vi "Individual curve visualization-Original.vi"() -> ()   [LabVIEW 2016]
panel:
  out "Drag V 4":cluster{dbl[], "Drag R":dbl[]}(graph)={[1.0, 1.2, 1.4, 1.6, 1.8, 2.0, 2.2, 2.4000000000000004, 2.6, 2.8, 3.0, 3.2, 3.4000000000000004, 3.6, 3.8000000000000003, 4.0, 4.2, 4.4, 4.6, 4.800000000000001, 5.0, 5.2, 5.4, 5.6000000000000005, 5.800000000000001, 6.0, 6.2, 6.4, 6.6000000000000005, 6.800000000000001, 7.0, 7.2, 7.4, 7.6000000000000005, 7.800000000000001, 8.0, 8.2, 8.4, 8.600000000000001, 8.8, 9.0], "Drag R"=[-3.300713023076663, -3.154449474386773, -1.6018811853832888, -1.623056110644585, -2.807731924651278, -4.278396429154972, -4.279502183141707, -4.366286193642124, -1.4410534649772644, 0.15566028543242932, 1.6991261140725915, 1.5692536155403247, 2.8580510224343625, 1.8206622631926488, 1.065024446971932, 0.32155007033235866, 0.4290224922843568, -0.6739053828926125, -1.9963504895407167, -1.9615097922476261, -3.7035483297953604, -2.7529582838595164, -3.432489372671602, -2.673522191757494, -3.4326797147495465, -4.140057534177399, -4.516110550482156, -6.970872132203194, -8.198832275397276, -5.3032397571211645, -3.8902609432575925, -5.869261674603283, -9.2239063545535, -6.918059763808269, -7.5433263379328475, -5.669627470898903, -6.863865171357286, -6.912037847582487, -5.835029601349728, -6.006897427720724, -7.171526427705753]}
  out "Drag V 2":cluster{dbl[], "Drag R":dbl[]}(graph)={[-1.0, -1.2, -1.4, -1.6, -1.8, -2.0, -2.2, -2.4000000000000004, -2.6, -2.8, -3.0, -3.2, -3.4000000000000004, -3.6, -3.8000000000000003, -4.0, -4.2, -4.4, -4.6, -4.800000000000001, -5.0, -5.2, -5.4, -5.6000000000000005, -5.800000000000001, -6.0, -6.2, -6.4, -6.6000000000000005, -6.800000000000001, -7.0, -7.2, -7.4, -7.6000000000000005, -7.800000000000001, -8.0, -8.2, -8.4, -8.600000000000001, -8.8, -9.0], "Drag R"=[-3.2437419601821214, -3.0741664524350005, -1.6279568878167145, -1.6200422715203617, -2.6283908576894714, -3.888715770646895, -3.977618456971424, -4.319620743435273, -1.3664134385707647, 0.320047182291161, 1.7072885590830775, 1.7630417095507562, 3.480405410849366, 1.8585977537912803, 1.1069080457471894, 0.19196943000107664, 0.36263224393675075, -0.5459969964599499, -2.246495774976516, -1.9887416826811497, -3.328699227235056, -2.8303882648843945, -3.046031238207835, -3.1669715718770597, -2.935142589811789, -4.499040388432356, -4.461115990090428, -6.5530890706250915, -7.938589412259593, -4.850132199040752, -3.8820527919237495, -5.861039921112386, -8.632298570084401, -6.880111107470923, -7.4081336329075675, -5.545023198155025, -6.610745934318789, -6.902518778616165, -5.879443445946976, -5.861498347694719, -7.106378902925503]}
  out "Drag V 3":cluster{dbl[], "Drag R":dbl[]}(graph)={[-1.0, -1.2, -1.4, -1.6, -1.8, -2.0, -2.2, -2.4000000000000004, -2.6, -2.8, -3.0, -3.2, -3.4000000000000004, -3.6, -3.8000000000000003, -4.0, -4.2, -4.4, -4.6, -4.800000000000001, -5.0, -5.2, -5.4, -5.6000000000000005, -5.800000000000001, -6.0, -6.2, -6.4, -6.6000000000000005, -6.800000000000001, -7.0, -7.2, -7.4, -7.6000000000000005, -7.800000000000001, -8.0, -8.2, -8.4, -8.600000000000001, -8.8, -9.0], "Drag R"=[8.506268720241243, 8.453111299769647, 5.837640325861369, 7.148519535853817, 5.613151260951883, 7.15271594863945, 6.035303430479679, 4.099468581977172, 3.8085835691967307, 2.146728062452322, 2.5912692993997513, 3.2852570243268238, 6.045815515529311, 5.520600455246357, 9.329259679090598, 10.480605588956307, 7.047030330219627, 8.091806546725207, 12.243345671940846, 13.329586545967194, 9.70803891981146, 10.868730098486818, 11.122912960745628, 10.009136477603038, 9.624346942261845, 8.817803908300313, 9.52354730833524, 6.612316030305441, 4.372195049370224, 2.659259797064494, 1.5932641526471045, 1.3933543185710036, 4.119548088345109, 5.4968037601237425, 6.930305725770583, 5.8104621629971245, 6.426504856124536, 6.12416493376701, 6.3797355980905195, 7.247784092040921, 6.868995388580276]}
  out "Drag R from V3":dbl[][](graph)=[[100.0], [100.0], [100.0], [100.0], [100.0], [100.0], [100.0], [100.0], [100.0], [100.0], [100.0], [100.0], [1.7525787802191088], [1.7024277791309896], [1.6796467941372961], [1.6622332596780016], [1.6326384430038565], [1.6030538217028973], [1.5750233368612336], [1.5464672130079027], [1.515305674671948], [1.4769663724594069], [1.4223433405393917], [1.367127876528625], [1.3303848800977325], [1.3258115595086495], [1.3319441343876612], [1.3412111211499946], [1.3504840018871018], [1.3569460556411512], [1.3612603273002564], [1.3655187586981927], [1.3717149148393943], [1.3853607545603541], [1.4256734959642343], [1.4882323948260159], [1.5646664564337707], [1.6600043991998266], [1.825179103810554], [2.0113113690130784], [2.153778457836145], [2.2061854757169623], [2.236759390639608], [2.2591165259970976], [2.271254546163343], [2.255116888990723], [2.131284142338929], [1.9300209107430364], [1.6997469455502165], [1.4689595661227408], [1.1719038462170055], [0.8507746640096665], [0.5682848756976853], [0.36799449880168633], [0.18504407697053282], [0.030652355361287242], [-0.06621522446930839], [-0.0895003694716015], [-0.09847025618305347], [-0.10464033846391654], [-0.10781778022866328], [-0.09364334174838697], [0.005606370088155135], [0.15965049598821562], [0.3473966553463515], [0.6442898471825012], [0.9527207762518782], [1.1676473220636312], [1.3374546714193756], [1.478434752127217], [1.5901322848992354], [1.6761660916131926], [1.7571344209049884], [1.8539291022681812], [1.9672049616575058], [2.084724071244043], [2.1942627160586827], [2.286993956635236], [2.37381081162657], [2.4528785475558], [2.5192696643991765], [2.570526739598677], [2.616689286852219], [2.6556743975271786], [2.682945368739358], [2.6962103781729607], [2.7059545183791447], [2.713853497772562], [2.719510645535571], [2.7225292908505287], [2.710925280793093], [2.6300724971380625], [2.507075147000063], [2.382324413515172], [2.284609434023482], [2.17962607717798], [2.0831734899557364], [2.022088082940096], [2.013507711742533], [2.0156321567498408], [2.0189057281954095], [2.022310702355015], [2.024991414457769], [2.0273587980551864], [2.029723297463262], [2.03228399843974], [2.0350593304874858], [2.037491663799248], [2.0404356617865664], [2.0449630021118885], [2.0589709240612515], [2.1147157107984738], [2.1951299818846985], [2.2809633053678966], [2.3878215220763006], [2.5123411459049585], [2.646121499165556], [2.7849929260300934], [2.94150608367427], [3.1001579479531576], [3.2446358461914926], [3.3828302948475217], [3.510267351861236], [3.6279185045827487], [3.738281105160597], [3.752281712877838], [3.716968130527663], [3.668561387705247], [3.6302480115875677], [3.619709418125278], [3.6170633689313596], [3.614338362318714], [3.6039982532236], [3.5632666463112197], [3.496188667064237], [3.4112673848251758], [3.302064135284801], [3.113108995158534], [2.9035833460838285], [2.7395191524712423], [2.6003692519174293], [2.470750349283642], [2.342683551892261], [2.2113055620953066], [2.084513208934559], [1.9502420264794773], [1.7841432231673235], [1.5808808468002922], [1.4589808708783767], [1.386113150959947], [1.3097468509102916], [1.2294193993280012], [1.3183489806063184], [1.7735900985853585], [1.8434364938950272], [1.6547838114359072], [1.4438849144543546], [1.1713380909804658], [0.9591404583844942], [0.9332570698213668], [0.9796520082449389], [1.0260469466685094], [1.0324380863668592], [1.0211745682940934], [1.0041594665245963], [0.9871443647550996], [0.9758808466823338], [0.9776632604651697], [1.0017554362928947], [1.0407717416081217], [1.0851455193601809], [1.1253101124984026], [1.1548084930482103], [1.1846991314501096], [1.2135526797068725], [1.2370487555268035], [1.250866976618206], [1.250745581339546], [1.2356121483481992], [1.2086064106811254], [1.1731312848415776], [1.132589687332811], [1.09038453465808], [1.0486634617941106], [1.001886957066429], [0.9485974335154795], [0.8884358369283974], [0.8210431130923201], [0.7460602077943783], [0.6601291617269677], [0.5483458064502711], [0.41616454664051356], [0.2724218383288142], [0.12595413754630536], [-0.014402099675880353], [-0.143103745292994], [-0.2729409413039015], [-0.40314083661617306], [-0.5298446554967583], [-0.6491936222126193], [-0.757328961030706], [-0.8530136281214128], [-0.9476966326108381], [-1.039060936123331], [-1.1221208120951789], [-1.19189053396267], [-1.2433843751620999], [-1.274731627175126], [-1.301236592248865], [-1.3251172476858604], [-1.3456543216920223], [-1.362128542473259], [-1.3738206382354787], [-1.3800113371845906], [-1.3804558837599505], [-1.3779361904824217], [-1.373879057238943], [-1.3693094440068145], [-1.3652523107633359], [-1.3627326174858072], [-1.3650331323236395], [-1.38469300364413], [-1.4198004223987497], [-1.4659599201843385], [-1.5187760285977352], [-1.573853279235783], [-1.626796203695321], [-1.6769446709488391], [-1.740232688366131], [-1.8106780565794993], [-1.8783318445699293], [-1.9332451213184072], [-1.965468955805924], [-1.9678038585291104], [-1.9512967158820373], [-1.920245912954881], [-1.8767003009131922], [-1.8227087309225247], [-1.7603200541484314], [-1.6915831217564676], [-1.6113302167838213], [-1.4819493743337553], [-1.3075715032524697], [-1.099948368593185], [-0.8708317354091007], [-0.6319733687534363], [-0.39512503367941276], [-0.16457147591045432], [0.0923245398572996], [0.37022252797865973], [0.656269081742926], [0.9376107944394273], [1.2013942593574631], [1.434766069786344], [1.6335917384754741], [1.8370718061323112], [2.040408441631051], [2.2300560533477376], [2.392469049658433], [2.5141018389391805], [2.581408829566029], [2.587269792136006], [2.563182205515298], [2.5186136886096357], [2.4573277088998084], [2.3830877338666054], [2.2996572309908103], [2.210799667753213], [2.1137606212460303], [1.976290685287626], [1.8035435235688344], [1.6075345200211748], [1.4002790585761735], [1.1937925231653364], [1.000090297720189], [0.82260339531407], [0.6252364316180199], [0.4200976984206837], [0.22825713135653058], [0.07078466606002365], [-0.031249761834372003], [-0.06770993281922782], [-0.09095212558221256], [-0.11083457660248139], [-0.12715113040549347], [-0.13969563151670594], [-0.14826192446157663], [-0.1526438537655633], [-0.14512720156245154], [-0.0859364276435621], [0.018640823505575527], [0.1542000683837651], [0.30633682348982466], [0.46064660532255874], [0.6027249303807714], [0.7264653052044163], [0.8673965864580044], [1.0197838582519936], [1.1696103702022502], [1.3028593719246406], [1.405514113035026], [1.4635578431492866], [1.4713967826342518], [1.4708139625800953], [1.4696628267175604], [1.4679585099118064], [1.4657161470279927], [1.4629508729312792], [1.4596778224868248], [1.455912130559789], [1.4485516507878464], [1.4207008268694026], [1.3738396138374274], [1.3127644697521716], [1.242271852673886], [1.1671582206628266], [1.0922200317792337], [1.022253744083363], [0.959672974401438], [0.8939020095272481], [0.8246069275278078], [0.7537171894972365], [0.6831622565296582], [0.614871589719183], [0.550774650159935], [0.4928008989460335], [0.4428797971715981], [0.4013447226544859], [0.3603397198822643], [0.31966426780318175], [0.2806907156474203], [0.24479141264515478], [0.21333870802656751], [0.18770495102183835], [0.16926249086114714], [0.1593836767746737], [0.15886460367700045], [0.16482085143572592], [0.1760060038779972], [0.19166109431666914], [0.21102715606459688], [0.23334522243463546], [0.25785632673964], [0.2838015022924656], [0.3104217824059673], [0.3382548894224496], [0.3738794064184983], [0.41670200668102686], [0.4647834984216126], [0.516184689851833], [0.5689663891832655], [0.6211894046274875], [0.6709145443960733], [0.7168732647431969], [0.7618980836377554], [0.8066315567273659], [0.8511286828950316], [0.895444461023756], [0.9396338899965421], [0.9837519686963905], [1.0278536960063103], [1.0719940708093016], [1.116115336607255], [1.1597000030691473], [1.202956201549208], [1.2462163791241851], [1.2898129828708271], [1.3340784598658797], [1.379345257186097], [1.4256277248076368], [1.471485296017775], [1.5172787744285805], [1.5637021239542714], [1.611449308509066], [1.661214292007178], [1.7136910383628323], [1.7695735114902438], [1.8309839883668162], [1.9046172824357102], [1.9860303747238839], [2.0690664855450898], [2.147568835213081], [2.215380644041606], [2.2686544985483668], [2.3172066161165055], [2.362599182869531], [2.404320218709873], [2.441857743539961], [2.4746997772622246], [2.5023343397790923], [2.525058473852339], [2.5470074952941992], [2.567949852570494], [2.586821988927007], [2.6025603476095247], [2.6141013718638315], [2.620381504935713], [2.6178575569635028], [2.594543402738337], [2.557003662884257], [2.514722061153872], [2.477182321299792], [2.4538681670746265], [2.450996819724539], [2.4547599206884096], [2.461936852620605], [2.472163159873596], [2.485074386799855], [2.500306077751855], [2.517493777082067], [2.541823826637785], [2.600923739891003], [2.6864026626294564], [2.783728630273892], [2.8783696782450603], [2.955793841963711], [3.0014691568505936], [3.007738172514057], [3.0067715943183995], [3.0048540219622972], [3.0020017170477096], [2.9982309411765975], [2.9935579559509216], [2.987999022972642], [2.973414339278415], [2.904782397172163], [2.7839265288191064], [2.621259310737942], [2.427193319447388], [2.2121411314661588], [1.9865153233129669], [1.7481776221828689], [1.4370709950539666], [1.0634145232580363], [0.6505154137173521], [0.22168087335410447], [-0.199781890909434], [-0.5982712108318664], [-1.0035001233111378], [-1.4172115456511012], [-1.8341969688897715], [-2.249247884065137], [-2.6571557822152676], [-3.052712154378151], [-3.4398842877940368], [-3.8581720136922337], [-4.28510172470091], [-4.68787441313243], [-5.033691071299138], [-5.289752691513447], [-5.440350650806982], [-5.5662261660846895], [-5.679776400419057], [-5.777530122860715], [-5.856016102460291], [-5.911763108268416], [-5.941299909335716], [-5.936400757868801], [-5.871887982418222], [-5.756966412187664], [-5.606353244398619], [-5.434765676272584], [-5.256920905031052], [-5.078369089309328], [-4.859207835558015], [-4.605965162097498], [-4.334378641472833], [-4.060185846229073], [-3.799124348911274], [-3.5600243887590945], [-3.315477715068531], [-3.069965462792207], [-2.834687008697351], [-2.6208417295512425], [-2.439629002121144], [-2.2951588654826103], [-2.155543185831086], [-2.023482653164767], [-1.9087060191267227], [-1.8209420353599974], [-1.7699194535076614], [-1.7588434198871203], [-1.7546606014535835], [-1.7512727653155618], [-1.7487007891590096], [-1.7469655506698811], [-1.7460879275341306], [-1.751855458263503], [-1.7936825787784874], [-1.8640515659725108], [-1.94909954627763], [-2.0349636461259024], [-2.1107657071835297], [-2.1861503338360158], [-2.2645484000403884], [-2.3470281963582473], [-2.434658013351197], [-2.5285061415808414], [-2.633447831862587], [-2.76576525688769], [-2.9108401979112632], [-3.049399933779855], [-3.1621717433399823], [-3.2372201905266857], [-3.3041944651830177], [-3.363676754655715], [-3.4094562056991617], [-3.4353219650677413], [-3.4354093432619446], [-3.4100311479385788], [-3.3646864233529454], [-3.3050221253948866], [-3.2366852099542447], [-3.157410520087679], [-3.033190405000106], [-2.8817392207732864], [-2.7295521108014844], [-2.590179295629865], [-2.4313802714044446], [-2.3150918660558855], [-2.3130125039363834], [-2.425028818075278], [-2.606877496788717], [-2.8722725286059783], [-3.327858992828627], [-3.5688180648142787], [-3.7199668472843137], [-3.8101565478293744], [-3.765288778462918], [-3.409697192443322], [-2.96679199430353], [-2.6741029939543584], [-2.448920146122463], [-2.252319045044758], [-2.084091564551963], [-1.94537691470312], [-1.6968735048719377], [-1.293886787102919], [-1.4580039927133661], [-2.7229885215063963], [-3.728654949645486], [-4.525405046288279], [-4.639098086182561], [-4.46956993412352], [-4.208072423868329], [-3.902287561082815], [-3.4638730574051255], [-2.9985198915565334], [-2.5018614682929248], [-1.9869828598242254], [-1.4593775800740074], [-0.8707832293898149], [-0.3601316708142035], [-0.04943995450805877], [0.19629323636639384], [0.3507948582790463], [0.3380162987393554], [0.1161254986409278], [-0.17535228671281733], [-0.4025506122009139], [-0.6102714962103372], [-0.8010438345558084], [-0.9593066584794848], [-1.088135677620042], [-1.2063186055947464], [-1.3330973990654873], [-1.49370455119218], [-1.7053497458468536], [-1.8962169972012424], [-2.0017639876829647], [-2.076050790635698], [-2.1342272050896534], [-2.1774242008695355], [-2.206641323395504], [-2.224769072375174], [-2.2393187437991924], [-2.2582161776527747], [-2.291500907840678], [-2.3526117398782858], [-2.433266923925575], [-2.522274438668859], [-2.6176510564344566], [-2.750262465402251], [-2.884404748568754], [-2.9736990783630604], [-2.987016538674169], [-2.9868701783838003], [-2.9865783454859103], [-2.9861419662582533], [-2.979278268104357], [-2.9335910059997827], [-2.856354685647265], [-2.7617169585063355], [-2.656398344199613], [-2.5093599053719773], [-2.3257280117302135], [-2.117986853952131], [-1.8893782784491395], [-1.607550511810117], [-1.3028805487474227], [-0.9824579479639529], [-0.6354517643496308], [-0.579855452817553], [-0.6407153728110055], [-0.7437725343279338], [-0.9048365575977063], [-1.2553362874988296], [-1.6557051691660387], [-1.9557175645738285], [-2.2181944080310125], [-2.436394184721253], [-2.5910998420360447], [-2.73024945698041], [-2.8443994645533324], [-2.9118650897136553], [-2.9178661838259345], [-2.892982538232731], [-2.8501280690589894], [-2.796516155796167], [-2.7310891036650964], [-2.6204167857222087], [-2.4863979073377283], [-2.3602003525067876], [-2.2671538426013678], [-2.19014483701028], [-2.1206356877785804], [-2.0544544152560076], [-1.987020025520782], [-1.9162190383509248], [-1.8490026216374156], [-1.7932323558824346], [-1.7533642275345251], [-1.7180854727779578], [-1.6950700847375808], [-1.6974015702912149], [-1.7342024779298217], [-1.784616006204022], [-1.824445681719345], [-1.8353832658857139], [-1.8385671833127937], [-1.8412587788651278], [-1.8457017990214601], [-1.8518605983869163], [-1.8592343363340902], [-1.8674439269625895], [-1.8769720039864102], [-1.890856160010116], [-1.9050975063953381], [-1.9146405860914009], [-1.9102579085078448], [-1.8688279095700862], [-1.798925339458748], [-1.7140709923625235], [-1.6170415168737422], [-1.467181415798466], [-1.293560381117423], [-1.1371354262072777], [-1.0269245022843725], [-0.9240605507913129], [-0.8366322922367193], [-0.7837575427369969], [-0.7785726464057602], [-0.7954719089281913], [-0.8250141629137189], [-0.8627580820395703], [-0.9088427829311257], [-0.9843819487818842], [-1.0845884842201712], [-1.1998806677958647], [-1.324418201720993], [-1.473138994843593], [-1.6454955306516061], [-1.8374289898957854], [-2.0448805533269785], [-2.2637914016959293]]
  out "Drag R from V2":dbl[][](graph)
  out "Drag R from V1":dbl[][](graph)
  in  "Tab Control":enum32{"Drag R and 4T R", " Line cut"}(tab)=enum." Line cut"
  in  "Input figure":cluster{dbl[], dbl[]}[](graph)
  out "Mean vs Curve":cluster{dbl[], dbl[]}(graph)
  in  "Group #":i32=40
  out "Vdrag 2":cluster{dbl[], dbl[]}(graph)
  out "Waveform Chart":T1(graph)={"Cursor.Cursor Y"=0.0, "Cursor.Cursor X"=-0.25874524714828895}
  in  "Drag V from V2":dbl[][](graph)=array4000x21[84000 elements]
  out "Trans R":cluster{dbl[], "Drag R":dbl[]}(graph)={[0.0, 1.0, 2.0, 3.0, 4.0, 5.0, 6.0, 7.0, 8.0, 9.0, 10.0, 11.0, 12.0, 13.0, 14.0, 15.0, 16.0, 17.0, 18.0, 19.0, 20.0], "Drag R"=[-1.955347401627896e-09, -1.806100631310869e-09, -1.819256861909132e-09, -1.793918202877933e-09, -1.796137693351605e-09, -1.807304893356547e-09, -1.805964965823982e-09, -1.790778062482098e-09, -1.803301930276354e-09, -1.805645839843799e-09, -1.80723227272443e-09, -1.80892591294674e-09, -1.814540522067394e-09, -1.822515647659391e-09, -1.803009188438047e-09, -1.799050033580806e-09, -1.792529699393382e-09, -1.811107636544342e-09, -1.809941044213503e-09, -1.791835456408071e-09, -1.82116905369291e-09]}
  out "Idrive":cluster{dbl[], dbl[]}[](graph)
  in  "stop":bool
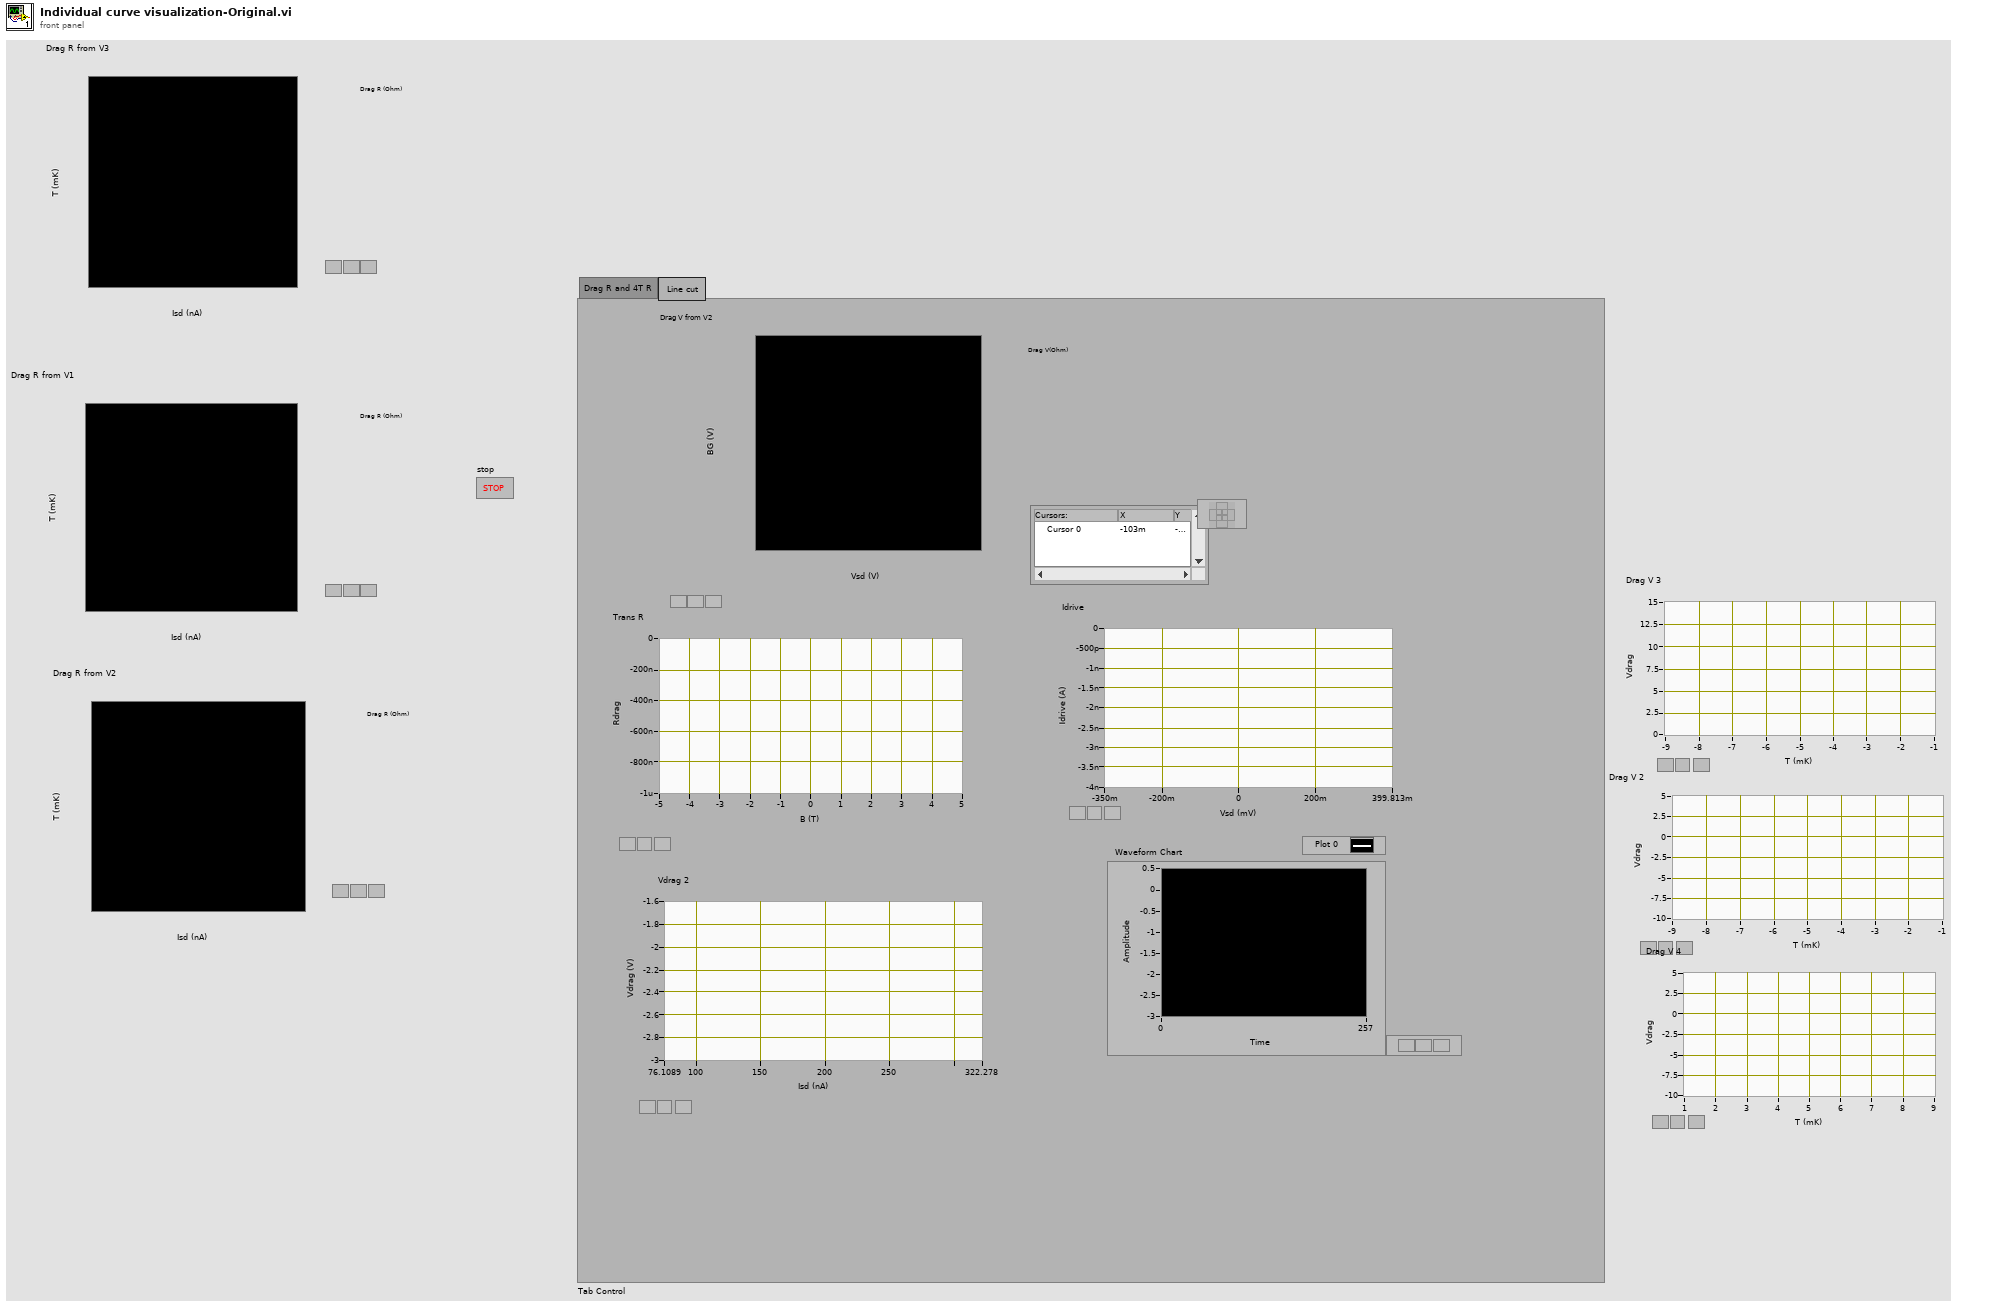
[diagram p1: front panel]
types:
  T1 = cluster{"Cursor.Cursor Y":dbl, "Cursor.Cursor X":dbl}
  T2 = typedef "LVOffsetAndMultiplierTypeDef.ctl" = cluster{"Offset":dbl, "Multiplier":dbl}
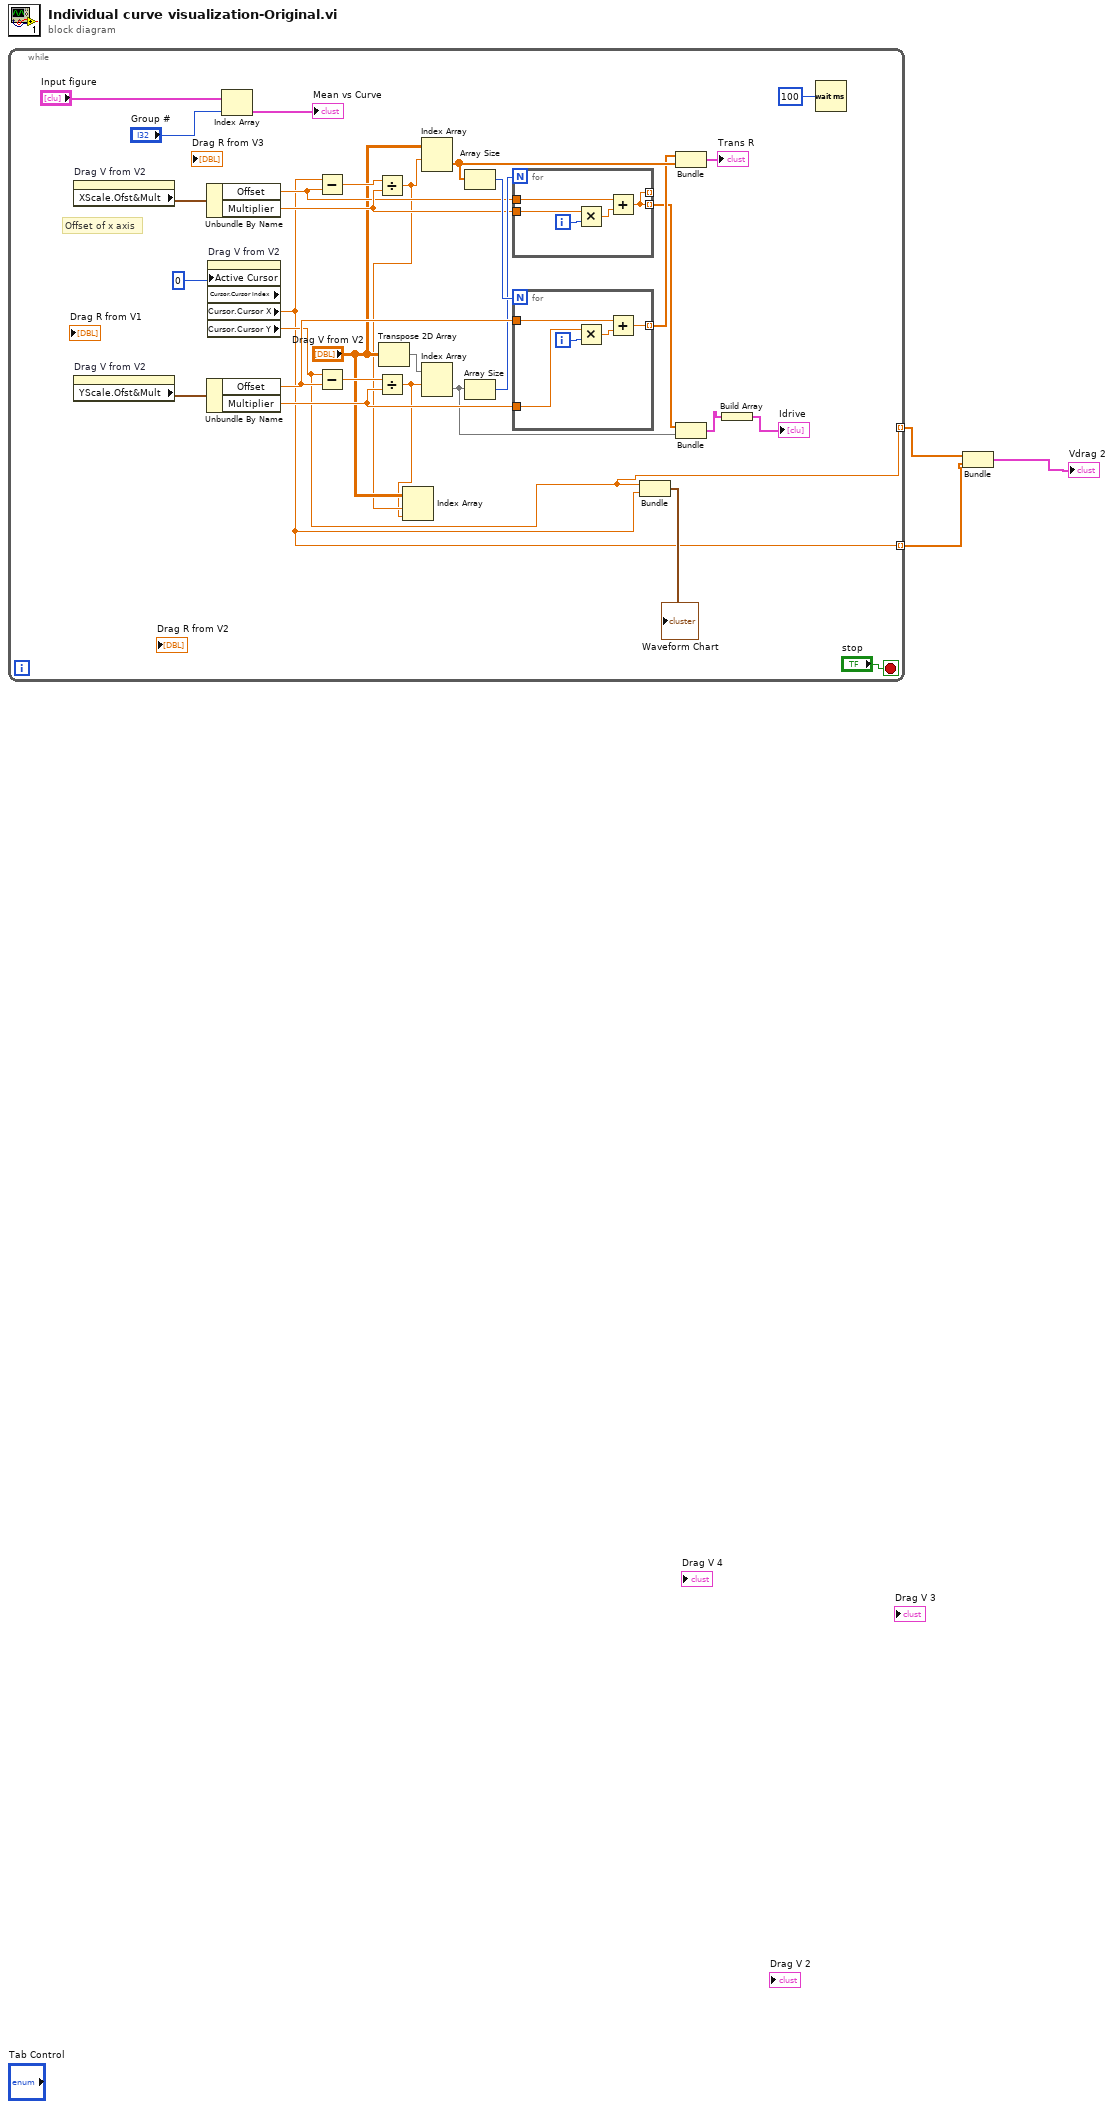
[diagram p0: block diagram]
diagram:
  n1 = while {
    tunnel: [w7] -> w3 mode=indexing
    tunnel: [w6] -> w2 mode=indexing
    stop <- "stop" stop-if-true
    # "Offset of x axis"
    n2 = property on="Drag V from V2" class="IntGraph (strict)"() -> ("XScale.Ofst&Mult"=w25:T2)  [unwired: 2 in, 2 out]
    n3 = property on="Drag V from V2" class="IntGraph (strict)"() -> ("YScale.Ofst&Mult"=w27:T2)  [unwired: 2 in, 2 out]
    n4 = Unbundle By Name(w25) -> ("Offset"=w15:dbl, "Multiplier"=w16:dbl)
    n5 = Unbundle By Name(w27) -> ("Offset"=w21:dbl, "Multiplier"=w23:dbl)
    n6 = property on="Drag V from V2" class="IntGraph (strict)" props=["Active Cursor", "Cursor", "Cursor Index", "Cursor", "Cursor X", "Cursor", "Cursor Y"]("Active Cursor"=u32 0) -> ("Cursor.Cursor X"=w6:dbl, "Cursor.Cursor Y"=w7:dbl)  [unwired: 2 in, 3 out]
    n7 = Index Array(array="Input figure", index="Group #") -> (element=→"Mean vs Curve":cluster{dbl[], dbl[]})
    n8 = Subtract(x=w6, y=w15) -> (x-y=w24:dbl)
    n9 = Subtract(x=w7, y=w21) -> (x-y=w26:dbl)
    n10 = Divide(x=w24, y=w16) -> (x/y=w11:dbl)
    n11 = Divide(x=w26, y=w23) -> (x/y=w10:dbl)
    n12 = Transpose 2D Array(2D array="Drag V from V2") -> (transposed array=w29:dbl[][])
    n13 = Index Array(array="Drag V from V2", index (row)=w11, index (col)=w10) -> ()  [unwired: 1 out]
    n14 = Index Array(array="Drag V from V2", index (row)=w11) -> (element=w20:dbl[])  [unwired: 1 in]
    n15 = Index Array(array=w29, index (row)=w10) -> (element=w18:dbl[])  [unwired: 1 in]
    n16 = Array Size(array=w20) -> (size(s)=w22:i32)
    n17 = Array Size(array=w18) -> (size(s)=w17:i32)
    n18 = for {
      N: w17 -> [_]
      tunnel: w16 -> [w37]
      tunnel: w15 -> [w35]
      tunnel: [w34] -> _ mode=indexing
      tunnel: [w34] -> w14 mode=indexing
      i -> [w38]
      n19 = Multiply(x=w37, y=w38) -> (x*y=w36:dbl)
      n20 = Add(x=w35, y=w36) -> (x+y=w34:dbl)
    }
    n21 = for {
      N: w22 -> [_]
      tunnel: w23 -> [w42]
      tunnel: w21 -> [w40]
      tunnel: [w39] -> w19 mode=indexing
      i -> [w43]
      n22 = Multiply(x=w42, y=w43) -> (x*y=w41:dbl)
      n23 = Add(x=w40, y=w41) -> (x+y=w39:dbl)
    }
    n24 = Bundle("Cursor.Cursor Y"=w7, "Cursor.Cursor X"=w6) -> (→"Waveform Chart":T1)  [unwired: 1 in]
    n25 = Bundle(w19, "Drag V from V2"=w20) -> (→"Trans R":cluster{dbl[], "Drag V from V2":dbl[]})  [unwired: 1 in]
    n26 = Bundle(w14, w18) -> (w5:cluster{dbl[], dbl[]})  [unwired: 1 in]
    n27 = Build Array(w5) -> (→"Idrive":cluster{dbl[], dbl[]}[])
    n28 = Wait (ms)(milliseconds to wait=u32 100) -> ()  [unwired: 1 out]
  }
  n29 = Bundle(w3, w2) -> (→"Vdrag 2":cluster{dbl[], dbl[]})  [unwired: 1 in]
